vi "daq.vi"() -> ()   [LabVIEW 2022 SP3]
panel:
  in  "Numeric 3":dbl
  in  "Numeric 2":dbl
  out "Numeric":dbl
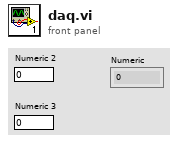
[diagram p1: front panel]
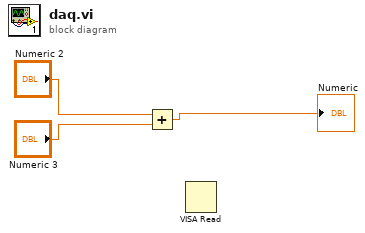
[diagram p0: block diagram]
diagram:
  n1 = Add(x="Numeric 2", y="Numeric 3") -> (x+y=→"Numeric":dbl)
  n2 = VISA Read() -> ()  [unwired: 3 in, 4 out]
